vi "Configure I2C.vi"(4 "SDA GPIO":T2=-1, 5 "Purpose (\"I2C\")":string="I2C", 6 "SCL GPIO":T2=-1, 7 "I2C #":T1=-1, 8 "error in (no error)":errorcluster, 10 "Baud":u32=400000 format="%.0p", 11 "Session in":refnum<class "Session.lvclass">) -> (0 "error out":errorcluster, 3 "Session out":refnum<class "Session.lvclass">)   [LabVIEW 2020, in "CTI.lvlib" / "Session.lvclass"]
uses:
  Session.lvclass
  GPIO Number.ctl
  I2C Number.ctl
  I2C Pins.ctl
  Session.lvclass/Session.ctl
  a62e29e6-9d1f-431a-a6fd-f8ae5f19d440.vi
  Is Full Errors.vi
  Check Errors.vi
  CTI.lvlib
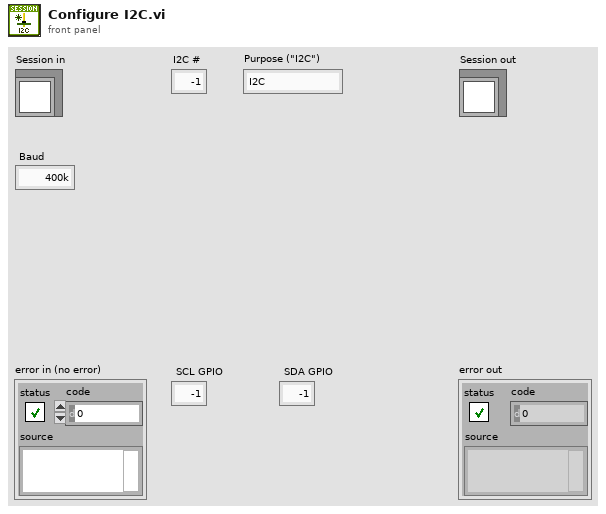
[diagram p1: front panel]
types:
  T1 = typedef "CTI.lvlib/I2C Number.ctl" = i8
  T2 = typedef "CTI.lvlib/GPIO Number.ctl" = i8
  T3 = typedef "CTI.lvlib/I2C Pins.ctl" = cluster{"SDA GPIO":T2, "SCL GPIO":T2}
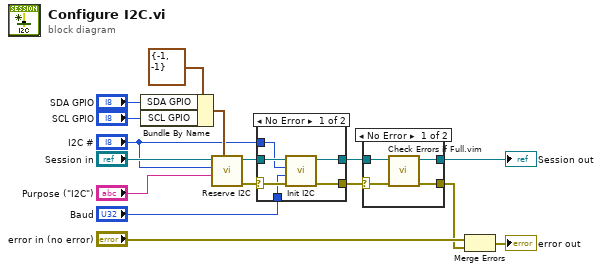
[diagram p0: block diagram]
diagram:
  n1 = Bundle By Name(cluster=T3 {"SDA GPIO"=-1, "SCL GPIO"=-1} ("I2C Pins"), "SDA GPIO"="SDA GPIO", "SCL GPIO"="SCL GPIO") -> (w13:T3)
  n2 = call "Reserve I2C.vi"("I2C Pins"=w13, "Purpose"="Purpose (\"I2C\")", "I2C #"="I2C #", "Session in"="Session in") -> ("error out"=w10:errorcluster, "Session out"=w9:refnum<class "Session.lvclass">)  [unwired: 6 in]
  n3 = case shown="No Error" w10 {
    selector: w10 -> [w21 w24]
    tunnel: w9 -> [w22 w23]
    tunnel: "Baud" -> [w20 _]
    tunnel: [w19 w23] -> w6
    tunnel: [w18 w24] -> w7
    tunnel: "I2C #" -> [w17 _]
    frame No Error {
      n4 = call-dynamic "Init I2C.vi"("error in (no error)"=w21, "Baud"=w20, "I2C In"=w17, "Session in"=w22) -> ("error out"=w18:errorcluster, "Session out"=w19:refnum<class "Session.lvclass">)  [unwired: 6 in]
    }
    frame Error {
    }
  }
  n5 = case shown="No Error" w7 {
    selector: w7 -> [w27 w29]
    tunnel: w6 -> [w28 w30]
    tunnel: [w26 w30] -> w5
    tunnel: [w25 w29] -> w3
    frame No Error {
      n6 = call "Check Errors if Full.vim"("error in (no error)"=w27, "Session in"=w28) -> ("error out"=w25:errorcluster, "Session out"=w26:refnum<class "Session.lvclass">)  [unwired: 8 in]
    }
    frame Error {
    }
  }
  "Session out" <- w5
  n7 = Merge Errors("error in (no error)", w3) -> (→"error out":errorcluster)
